vi "Read Lights and Append.vi"(0 "Input (Old) Light Sensor Array":i32[](array[numeric])=[1, 2, 3, 4, 5, 6, 7, 8, 9, 1, 2, 3, 4, 5, 6, 7, 8, 9]) -> (5 "Output Light Sensor Array":i32[](array[numeric]))   [LabVIEW 2018]
uses:
  <vilib>/myRIO/Instrument Drivers/Onboard IO/DIO/typedefs/DIO Reference.ctl
  <vilib>/myRIO/Common/Instrument Driver Framework/Utilities/typedefs/myRIO Generic Hardware Reference.ctl
  <vilib>/myRIO/Common/Instrument Driver Framework/Utilities/typedefs/Hardware Version Enum.ctl
  <vilib>/myRIO/Common/Instrument Driver Framework/Utilities/typedefs/myRIO v1.0 Reference.ctl
  <vilib>/myRIO/Common/Instrument Driver Framework/Utilities/typedefs/Generic FPGA Reference.ctl
  <vilib>/myRIO/Common/Instrument Driver Framework/myRIO v1.0/DIO/typedefs/DIO Channels List.ctl
  <vilib>/myRIO/Common/Instrument Driver Framework/myRIO v1.0/DIO/typedefs/DIO Channels Enum.ctl
  <vilib>/userdefined/High Color/nirio_resource_hc.ctl
  <vilib>/myRIO/Common/Instrument Driver Framework/Utilities/vis/Is FPGA Ref Available.vi
  <vilib>/myRIO/Common/Instrument Driver Framework/myRIO v1.0/DIO/vis/myRIO v1.1 Open DIO.vi
  <vilib>/myRIO/Instrument Drivers/Onboard IO/DIO/vis/Read.vi
  <vilib>/myRIO/Common/Instrument Driver Framework/Utilities/vis/Validate Channels.vi
  <vilib>/myRIO/Common/Instrument Driver Framework/myRIO v1.0/DIO/vis/myRIO v1.0 Reserve DIO.vi
  <vilib>/myRIO/Common/Instrument Driver Framework/myRIO v1.0/Resource Manager/vis/myRIO v1.0 Reserve Channel List.vi
  <vilib>/myRIO/Common/Instrument Driver Framework/myRIO v1.0/DIO/vis/myRIO v1.0 Build MUX Configuration DIO.vi
  <vilib>/myRIO/Common/Instrument Driver Framework/myRIO v1.0/Resource Manager/vis/myRIO v1.0 Reserve Channel.vi
  <vilib>/myRIO/Common/Instrument Driver Framework/myRIO v1.0/Resource Manager/vis/myRIO v1.0 Unreserve Channel.vi
  <vilib>/myRIO/Common/Instrument Driver Framework/myRIO v1.0/Resource Manager/vis/myRIO v1.0 Create Configuration List.vi
  <vilib>/myRIO/Common/Instrument Driver Framework/myRIO v1.0/Resource Manager/vis/myRIO v1.0 Build Mutex Name.vi
  <vilib>/Utility/VariantDataType/GetNumericInfo.vi
  <vilib>/Utility/error.llb/Error Cluster From Error Code.vi
  <vilib>/myRIO/Common/Instrument Driver Framework/myRIO v1.0/myRIO v1.1 Open.vi
  <vilib>/myRIO/Common/Instrument Driver Framework/Utilities/vis/IO Manager.vi
  <vilib>/myRIO/Common/Instrument Driver Framework/Utilities/vis/Configuration Manager.vi
  <vilib>/myRIO/Common/Instrument Driver Framework/myRIO v1.0/Resource Manager/vis/myRIO v1.0 Configure IO.vi
  <vilib>/myRIO/Common/Instrument Driver Framework/myRIO v1.0/myRIO v1.0 Close.vi
  <vilib>/myRIO/Common/Instrument Driver Framework/myRIO v1.0/DIO/vis/myRIO v1.0 Read DIO.vi
  <vilib>/myRIO/Express VI/Onboard IO/DI/DI Express VI.xnode
  <vilib>/myRIO/Instrument Drivers/Onboard IO/DIO/vis/myRIO DIO Open.xnode
  <vilib>/myRIO/Instrument Drivers/Onboard IO/DIO/DIO.lvlib
panel:
  out "B/DIO14 (Pin 32)":bool
  out "A/DIO14 (Pin 32)":bool
  out "A/DIO12 (Pin 22)":bool
  out "A/DIO15 (Pin 34)":bool
  out "A/DIO11 (Pin 18)":bool
  out "A/DIO10 (Pin 31)":bool
  out "A/DIO1 (Pin 13)":bool
  out "B/DIO15 (Pin 34)":bool
  out "A/DIO13 (Pin 26)":bool
  out "A/DIO9 (Pin 29)":bool
  out "A/DIO8 (Pin 27)":bool
  out "A/DIO5 (Pin 21)":bool
  out "A/DIO6 (Pin 23)":bool
  out "A/DIO7 (Pin 25)":bool
  out "A/DIO3 (Pin 17)":bool
  out "A/DIO2 (Pin 15)":bool
  out "A/DIO0 (Pin 11)":bool
  out "A/DIO4 (Pin 19)":bool
  out "appended array":bool[](array[boolean])
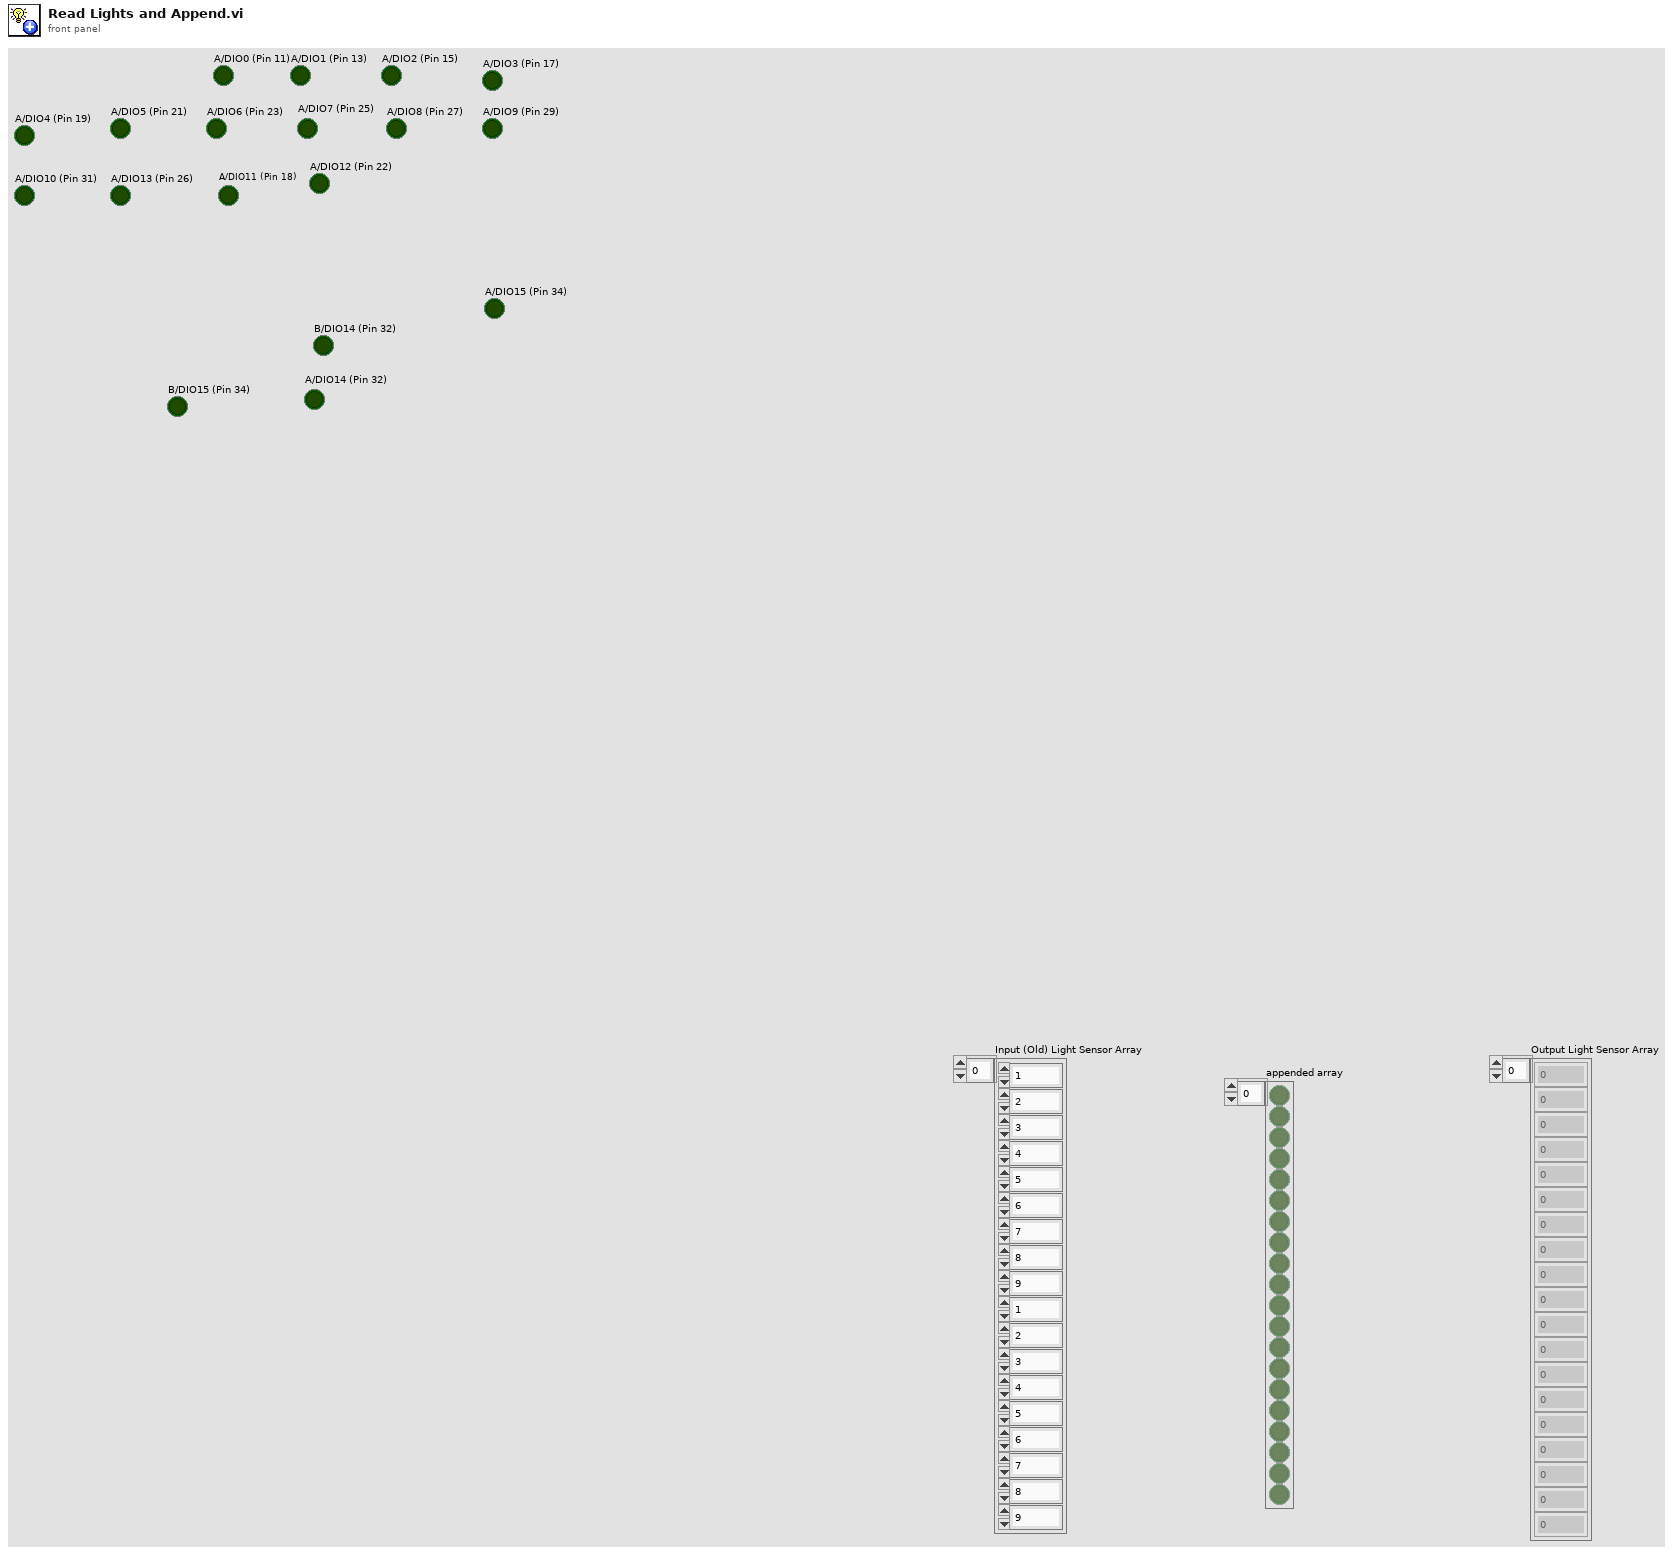
[diagram p1: front panel]
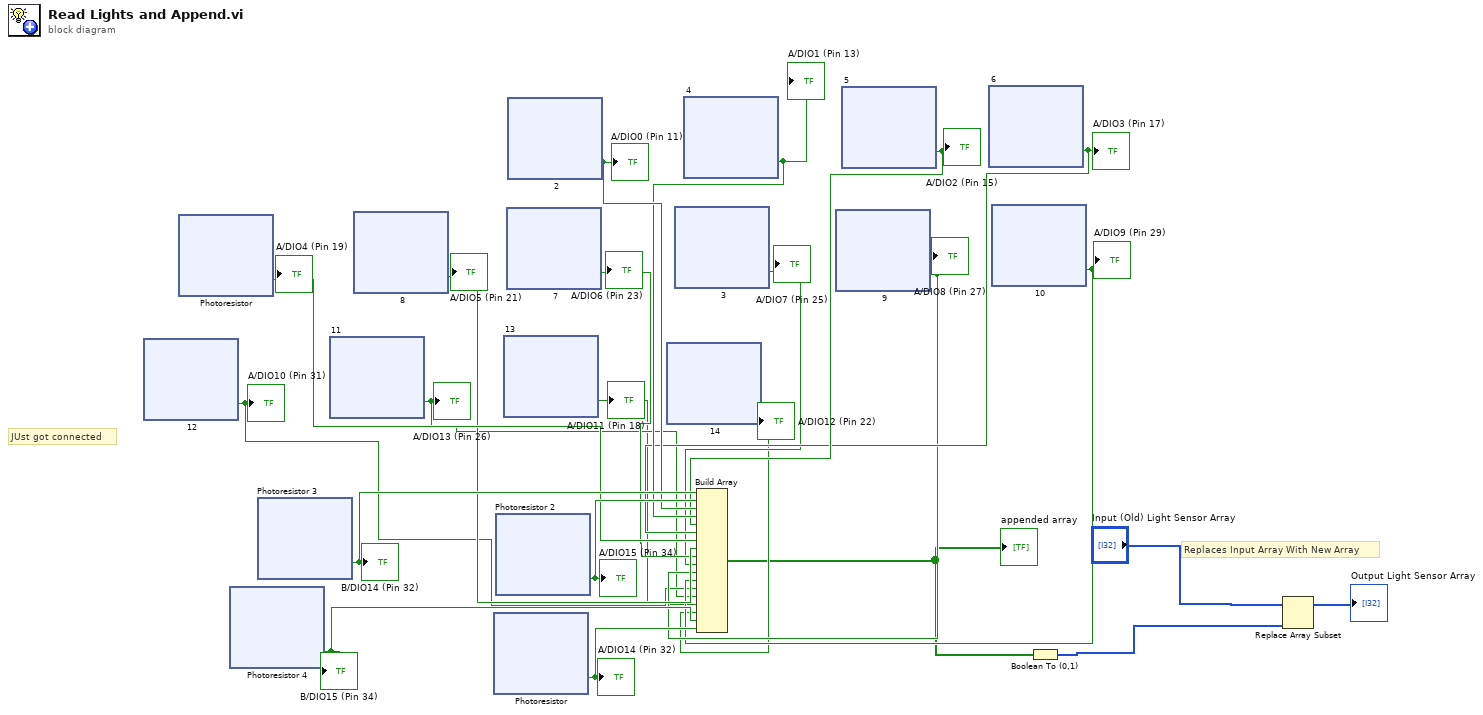
[diagram p0: block diagram]
diagram:
  # "JUst got connected"
  # "Replaces Input Array With New Array"
  n1 = xnode " 12"() -> ("A/DIO10 (Pin 31)"=w5:bool)  [unwired: 1 in, 1 out]
  "A/DIO10 (Pin 31)" <- w5
  n2 = xnode "Photoresistor"() -> ("A/DIO4 (Pin 19)"=w11:bool)  [unwired: 1 in, 1 out]
  "A/DIO4 (Pin 19)" <- w11
  n3 = xnode "Photoresistor 4"() -> ("B/DIO15 (Pin 34)"=w17:bool)  [unwired: 1 in, 1 out]
  "B/DIO15 (Pin 34)" <- w17
  n4 = xnode "Photoresistor 3"() -> ("B/DIO14 (Pin 32)"=w19:bool)  [unwired: 1 in, 1 out]
  "B/DIO14 (Pin 32)" <- w19
  n5 = xnode " 11"() -> ("A/DIO13 (Pin 26)"=w4:bool)  [unwired: 1 in, 1 out]
  "A/DIO13 (Pin 26)" <- w4
  n6 = xnode " 8"() -> ("A/DIO5 (Pin 21)"=w10:bool)  [unwired: 1 in, 1 out]
  "A/DIO5 (Pin 21)" <- w10
  n7 = xnode "Photoresistor"() -> ("A/DIO14 (Pin 32)"=w16:bool)  [unwired: 1 in, 1 out]
  "A/DIO14 (Pin 32)" <- w16
  n8 = xnode "Photoresistor 2"() -> ("A/DIO15 (Pin 34)"=w18:bool)  [unwired: 1 in, 1 out]
  "A/DIO15 (Pin 34)" <- w18
  n9 = xnode " 13"() -> ("A/DIO11 (Pin 18)"=w3:bool)  [unwired: 1 in, 1 out]
  "A/DIO11 (Pin 18)" <- w3
  n10 = xnode " 7"() -> ("A/DIO6 (Pin 23)"=w9:bool)  [unwired: 1 in, 1 out]
  "A/DIO6 (Pin 23)" <- w9
  n11 = xnode " 2"() -> ("A/DIO0 (Pin 11)"=w15:bool)  [unwired: 1 in, 1 out]
  "A/DIO0 (Pin 11)" <- w15
  n12 = xnode " 14"() -> ("A/DIO12 (Pin 22)"=w2:bool)  [unwired: 1 in, 1 out]
  "A/DIO12 (Pin 22)" <- w2
  n13 = xnode " 3"() -> ("A/DIO7 (Pin 25)"=w8:bool)  [unwired: 1 in, 1 out]
  "A/DIO7 (Pin 25)" <- w8
  n14 = xnode " 4"() -> ("A/DIO1 (Pin 13)"=w14:bool)  [unwired: 1 in, 1 out]
  "A/DIO1 (Pin 13)" <- w14
  n15 = xnode " 9"() -> ("A/DIO8 (Pin 27)"=w7:bool)  [unwired: 1 in, 1 out]
  "A/DIO8 (Pin 27)" <- w7
  n16 = xnode " 5"() -> ("A/DIO2 (Pin 15)"=w13:bool)  [unwired: 1 in, 1 out]
  "A/DIO2 (Pin 15)" <- w13
  n17 = xnode " 6"() -> ("A/DIO3 (Pin 17)"=w12:bool)  [unwired: 1 in, 1 out]
  "A/DIO3 (Pin 17)" <- w12
  n18 = xnode " 10"() -> ("A/DIO9 (Pin 29)"=w6:bool)  [unwired: 1 in, 1 out]
  "A/DIO9 (Pin 29)" <- w6
  n19 = Build Array(w19, w18, w15, w14, w13, w12, w11, w10, w9, w8, w7, w6, w5, w4, w3, w2, w17, w16) -> (w1:bool[])
  "appended array" <- w1
  n20 = Boolean To (0,1)(Boolean=w1) -> (0, 1=w20:i16[])
  n21 = Replace Array Subset(array="Input (Old) Light Sensor Array", new element=w20) -> (→"Output Light Sensor Array":i32[])  [unwired: 1 in]
